vi "Climb (SubVI).vi"(7 "At position and not third":bool, 8 "C":dbl, 9 "Arm Current":dbl, 10 "Solenoid in":T1, 11 "Input from Speed logic":dbl) -> (1 "Arm Motor":dbl, 2 "Arm Set":dbl, 3 "Solenoid out":T1)   [LabVIEW 2012]
uses:
  <vilib>/Rock Robotics/WPI/Solenoid/WPI_SolenoidValue.ctl
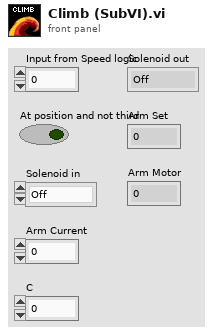
[diagram p1: front panel]
types:
  T1 = typedef "WPI_SolenoidValue.ctl" = enum16{"Off", "On", "Forward", "Reverse"}
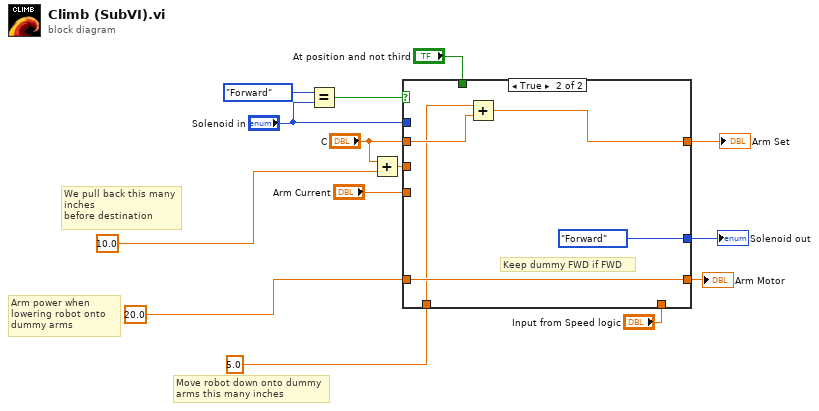
[diagram p0: block diagram]
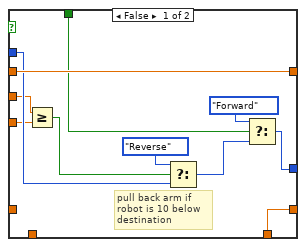
[diagram p2: hidden frame]
diagram:
  # "Move robot down onto dummy arms this many inches"
  # "Arm power when lowering robot onto dummy arms"
  # "We pull back this many inches\nbefore destination"
  n1 = Equal?(x=WPI_SolenoidValue."Forward" ("y"), y="Solenoid in") -> (x = y?=w4:bool)
  n2 = Add(x="C", y=10.0) -> (x+y=w10:dbl)
  n3 = case shown="True" w4 {
    tunnel: [w24 w29] -> w12
    tunnel: "C" -> [w24 w30]
    tunnel: [w23 WPI_SolenoidValue."Forward" ("Value")] -> w5
    tunnel: "Input from Speed logic" -> [w25 _]
    tunnel: [w25 w27] -> w7
    tunnel: "At position and not third" -> [w21 _]
    tunnel: w10 -> [w16 _]
    tunnel: "Arm Current" -> [w15 _]
    tunnel: "Solenoid in" -> [w17 _]
    tunnel: 20.0 ("f") -> [_ w27]
    tunnel: 5.0 ("x") -> [_ w26]
    frame False {
      # "pull back arm if robot is 10 below destination"
      n4 = Greater Or Equal?(x=w16, y=w15) -> (x >= y?=w18:bool)
      n5 = Select(t=WPI_SolenoidValue."Reverse" ("Value"), s=w18, f=w17) -> (s? t:f=w20:T1)
      n6 = Select(t=WPI_SolenoidValue."Forward", s=w21, f=w20) -> (s? t:f=w23:T1)
    }
    frame True {
      # "Keep dummy FWD if FWD"
      n7 = Add(x=w26, y=w30) -> (x+y=w29:dbl)
    }
  }
  "Arm Set" <- w12
  "Arm Motor" <- w7
  "Solenoid out" <- w5
